vi "PSTRA-Reprocess Raw Data File.vi"(0 "Path":path, 7 "Runtime in":T1 {"window" items=["None ", "Hanning", "Hamming", "Blackman-Harris", "Exact Blackman", "Blackman", "Flat Top", "4 Term B-Harris ", "7 Term B-Harris", "Low Sidelobe"]; "stimChan"."Filter"."Stages"."IIR Filter"."Forward Coefficients" format="%.4f"; "stimChan"."Filter"."Stages"."IIR Filter"."Reverse Coefficients" format="%.4f"}, 11 "error in (no error)":errorcluster) -> (4 "Runtime out":T1 {"window" items=["None ", "Hanning", "Hamming", "Blackman-Harris", "Exact Blackman", "Blackman", "Flat Top", "4 Term B-Harris ", "7 Term B-Harris", "Low Sidelobe"]; "stimChan"."Filter"."Stages"."IIR Filter"."Forward Coefficients" format="%.4f"; "stimChan"."Filter"."Stages"."IIR Filter"."Reverse Coefficients" format="%.4f"}, 6 "PSD":dbl[][](array[numeric]), 8 "PSTH":dbl[](array[numeric]), 10 "Amplitude":dbl, 15 "error out":errorcluster)   [LabVIEW 2020]
uses:
  Typedefs/PSTR-Runtime Data.ctl
  Signal Synthesis VIs/Controls/Stimulus Channel (Full)/Full Stimulus Channel Data.ctl
  Signal Synthesis VIs/Controls/Waveform XCtl/Waveform Data.ctl
  Signal Synthesis VIs/Controls/Waveform XCtl/Waveform Enum.ctl
  Signal Synthesis VIs/Waveform VIs/Tone VIs/Tone Params.ctl
  Signal Synthesis VIs/Waveform VIs/Pulse Train VIs/Pulse Train Params.ctl
  Signal Synthesis VIs/Waveform VIs/Pulse Train VIs/Pulse Polarity.ctl
  Signal Synthesis VIs/Waveform VIs/Pulse Train VIs/PT-Continuous State.ctl
  Signal Synthesis VIs/Waveform VIs/Noise VIs/Noise Params.ctl
  Signal Synthesis VIs/Waveform VIs/File VIs/StimFile-Params.ctl
  Signal Synthesis VIs/Waveform VIs/FM Sweep VIs/FM Sweep Params.ctl
  Signal Synthesis VIs/Waveform VIs/Chirp Train VIs/Chirp Train.ctl
  Signal Synthesis VIs/Waveform VIs/Chirp Train VIs/Chirp Train Params.ctl
  Signal Synthesis VIs/Waveform VIs/Complex Tone VIs/CT-Params.ctl
  Signal Synthesis VIs/Waveform VIs/Complex Tone VIs/CT-Phase Enum.ctl
  Signal Synthesis VIs/Waveform VIs/Complex Tone VIs/CT-Runtime Data.ctl
  Signal Synthesis VIs/Waveform VIs/Moving Ripple VIs/Moving Ripple.ctl
  Signal Synthesis VIs/Waveform VIs/Moving Ripple VIs/Moving Ripple.Params.ctl
  Signal Synthesis VIs/Waveform VIs/Moving Ripple VIs/Moving Ripple.Data.ctl
  Signal Synthesis VIs/Controls/Advanced Filter XCtl/Filter Data.ctl
  Signal Synthesis VIs/Filter VIs/Filter-Bandwidth Units.ctl
  Signal Synthesis VIs/Controls/Burst XCtl/Burst Data.ctl
  Signal Synthesis VIs/Controls/Level XCtl/Level Data.ctl
  Signal Synthesis VIs/Controls/Level XCtl/Level Units.ctl
  Signal Synthesis VIs/Controls/Advanced Options XCtl/Advanced Stimulus Options.ctl
  Signal Synthesis VIs/Modulation VIs/SAM VIs/SAM Params.ctl
  <vilib>/addons/Time Series Analysis/Correlation and Spectral Analysis.llb/TSA Welch (Array).vi
  <vilib>/addons/_Advanced Signal Processing/NI_AdvSigProcTSA.lvlib
panel:
  out "reject":bool
  in  "Override":bool=TRUE
  in  "RejThr":dbl
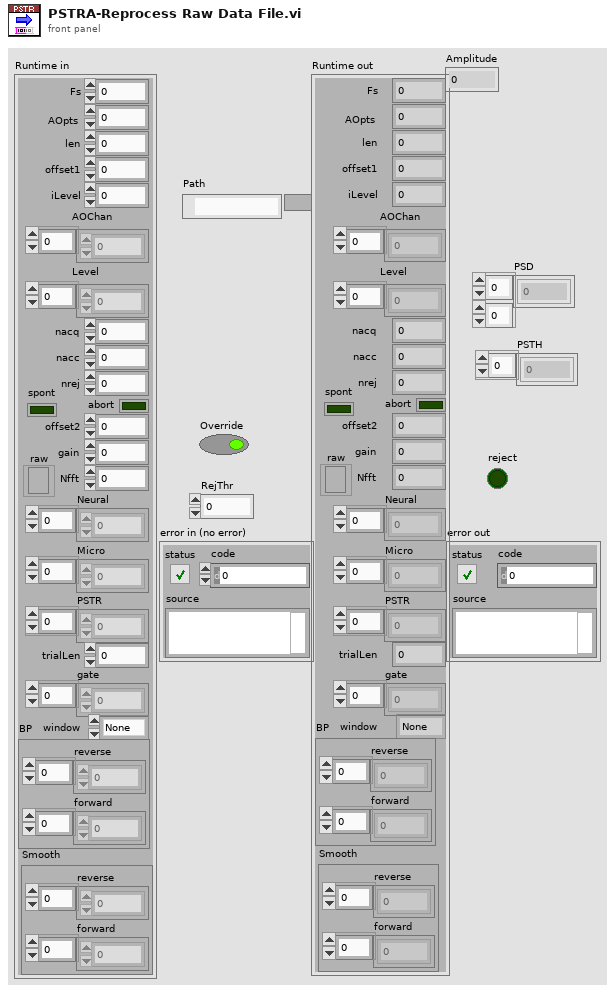
[diagram p1: front panel]
types:
  T1 = typedef "PSTR-Runtime Data.ctl" = cluster{"Fs":dbl, "AOpts":i32, "stimChan":T2, "len":i32, "offset1":i32, "iLevel":i32, "AOChan":i32[], "Level":dbl[], "nacc":i32, "nrej":i32, "nacq":i32, "abort":bool, "offset2":i32, "gain":dbl, "Nfft":i32, "Neural":dbl[], "Micro":dbl[], "raw":refnum<file>, "spont":bool, "PSTR":dbl[], "trialLen":i32, "gate":dbl[], "window":u16, "BP":cluster{"reverse":dbl[], "forward":dbl[]}, "Smooth":cluster{"reverse":dbl[], "forward":dbl[]}}
  T2 = typedef "Stimulus Channel (Full).xctl/Full Stimulus Channel Data.ctl" = cluster{"Waveform":T3, "Filter":T20, "Burst":T22, "Level":T23, "Name":string, "Advanced":T25, "SAM":T26}
  T3 = typedef "Waveform XCtl.xctl/Waveform Data.ctl" = cluster{"Type":T4, "Tone":T5, "Pulse Train":T6, "Noise":T9, "File":T10, "FMSweep":T11, "Chirp Train":T12, "Complex Tone":cluster{"Params":T14, "Data":T16}, "Moving Ripple":T17}
  T4 = typedef "Waveform Enum.ctl" = enum16{"OFF", "Tone", "Noise", "Pulse Train", "File", "FM Sweep", "Chirp Train", "Complex Tone", "FM Tone", "Moving Ripple"}
  T5 = typedef "Tone Params.ctl" = cluster{"Frequency (kHz)":dbl, "Last Freq":dbl, "Last Phase":dbl}
  T6 = typedef "Pulse Train Params.ctl" = cluster{"Pulse width (us)":dbl, "Pulse rate (Hz)":dbl, "Gap (ms)":dbl, "Polarity":T7, "PT State":T8, "Asynch":bool}
  T7 = typedef "Pulse Polarity.ctl" = enum16{"POS", "NEG", "POS-NEG", "NEG-POS"}
  T8 = typedef "PT-Continuous State.ctl" = cluster{"Template":dbl[], "Nperiod":i32, "Index":i32, "Pulse Rate (Hz)":dbl, "Phase (cycles)":dbl, "Noff":i32}
  T9 = typedef "Noise Params.ctl" = cluster{"InvFilt":bool, "Noise":dbl[], "CurPt":i32, "Aweight":bool, "Seed":i32, "afile":path}
  T10 = typedef "StimFile-Params.ctl" = cluster{"Filename":path, "Signal":dbl[], "Channel":i32, "stream":bool, "offset":i32, "nreps":i32, "loops":i32, "Randomize":bool, "order":i32[], "Seed":i32, "Tokens":i32}
  T11 = typedef "FM Sweep Params.ctl" = cluster{"Rate (oct/s)":dbl, "Fmin (Hz)":dbl, "Fmax (Hz)":dbl, "Ramp (ms)":dbl, "Linear":bool}
  T12 = typedef "Chirp Train.ctl" = cluster{"Params":T13, "Data":cluster{"WF":dbl[]}}
  T13 = typedef "Chirp Train Params.ctl" = cluster{"Fmin (kHz)":dbl, "Fmax (kHz)":dbl, "Compensate":bool, "Duration (ms)":dbl}
  T14 = typedef "CT-Params.ctl" = cluster{"F0 (Hz)":dbl, "Band":cluster{"Flow (Hz)":dbl, "Fhigh (Hz)":dbl}, "Phase":T15, "Min F0 (Hz)":dbl, "Max F0 (Hz)":dbl, "ContinRandPhase":bool, "Max peak factor":dbl, "Max mod depth":dbl, "MinHarmNum":i32, "MaxHarmNum":i32, "Level Mode":enum16{"per component", "overall rms"}, "% jitter":dbl}
  T15 = typedef "CT-Phase Enum.ctl" = enum16{"Cosine", "Random", "Alternating"}
  T16 = typedef "CT-Runtime Data.ctl" = cluster{"Ncomp":i32, "MinHarm":i32, "Phase":dbl[], "Amplitude":dbl[], "Npts/frame":i32, "Last F0":dbl, "Fmin":dbl, "Fmax":dbl, "Lslope":dbl, "randphase":bool, "overall rms":bool, "fmult":dbl[], "jittered":bool}
  T17 = typedef "Moving Ripple.ctl" = cluster{"Params":T18, "Data":T19}
  T18 = typedef "Moving Ripple.Params.ctl" = cluster{"Fmin":dbl, "Fmax":dbl, "Density":dbl, "Velocity":dbl, "Depth":dbl, "Phase":dbl, "Comp/oct":i32}
  T19 = typedef "Moving Ripple.Data.ctl" = cluster{"Freq":dbl[], "A":dbl[], "phase":dbl[], "Phase":dbl}
  T20 = typedef "Advanced Filter XCtl.xctl/Filter Data.ctl" = cluster{"Type":enum16{"Lowpass", "Highpass", "Bandpass", "Bandstop", "OFF"}, "CF (kHz)":dbl, "BW (kHz)":dbl, "Cascade":bool, "Quadrature":bool, "Scale Factor":dbl, "Stages":cluster{"IIR Filter":cluster{"filter structure":enum32{"IIR 2nd Order", "IIR 4th Order"}, "Reverse Coefficients":dbl[], "Forward Coefficients":dbl[]}, "State":dbl[]}[], "Class":enum16{"Elliptic", "Butterworth"}, "Order":i32, "BWUnits":T21}
  T21 = typedef "Filter-Bandwidth Units.ctl" = enum16{"Linear", "Octaves", "Min-Max"}
  T22 = typedef "Burst Control.xctl/Burst Data.ctl" = cluster{"Active":bool, "Delay (ms)":dbl, "Duration (ms)":dbl, "Ramp (ms)":dbl, "Rate (Hz)":dbl, "Trepeat (ms)":dbl, "Repeat":bool}
  T23 = typedef "Level XCtl.xctl/Level Data.ctl" = cluster{"Level":dbl, "Units":T24, "Max":dbl, "Multiplier":dbl, "Cal File":path, "Cal":cluster{"Freq (Hz)":dbl[], "Mag (dB SPL)":dbl[], "Phase (deg)":dbl[]}}
  T24 = typedef "Level Units.ctl" = enum16{"dB atten", "dB SPL", "dB re 1 Vrms", "dB V/Hz½", "mW", "dB HL", "Volts", "dB mW"}
  T25 = typedef "Advanced Stimulus Options.xctl/Advanced Stimulus Options.ctl" = cluster{"Rep Mask":string, "AltPol":bool, "Var":string, "Expr":string, "Persist":bool}
  T26 = typedef "SAM Params.ctl" = cluster{"Active":bool, "Frequency (Hz)":dbl, "Depth":dbl, "Init Phase (cycles)":dbl, "phase (degrees)":dbl, "Asynch":bool}
  T27 = enum16{"open", "replace", "create", "open or create", "replace or create", "replace or create with confirmation"}
  T28 = cluster{"window":u16, "length":i32, "overlap (%)":dbl}
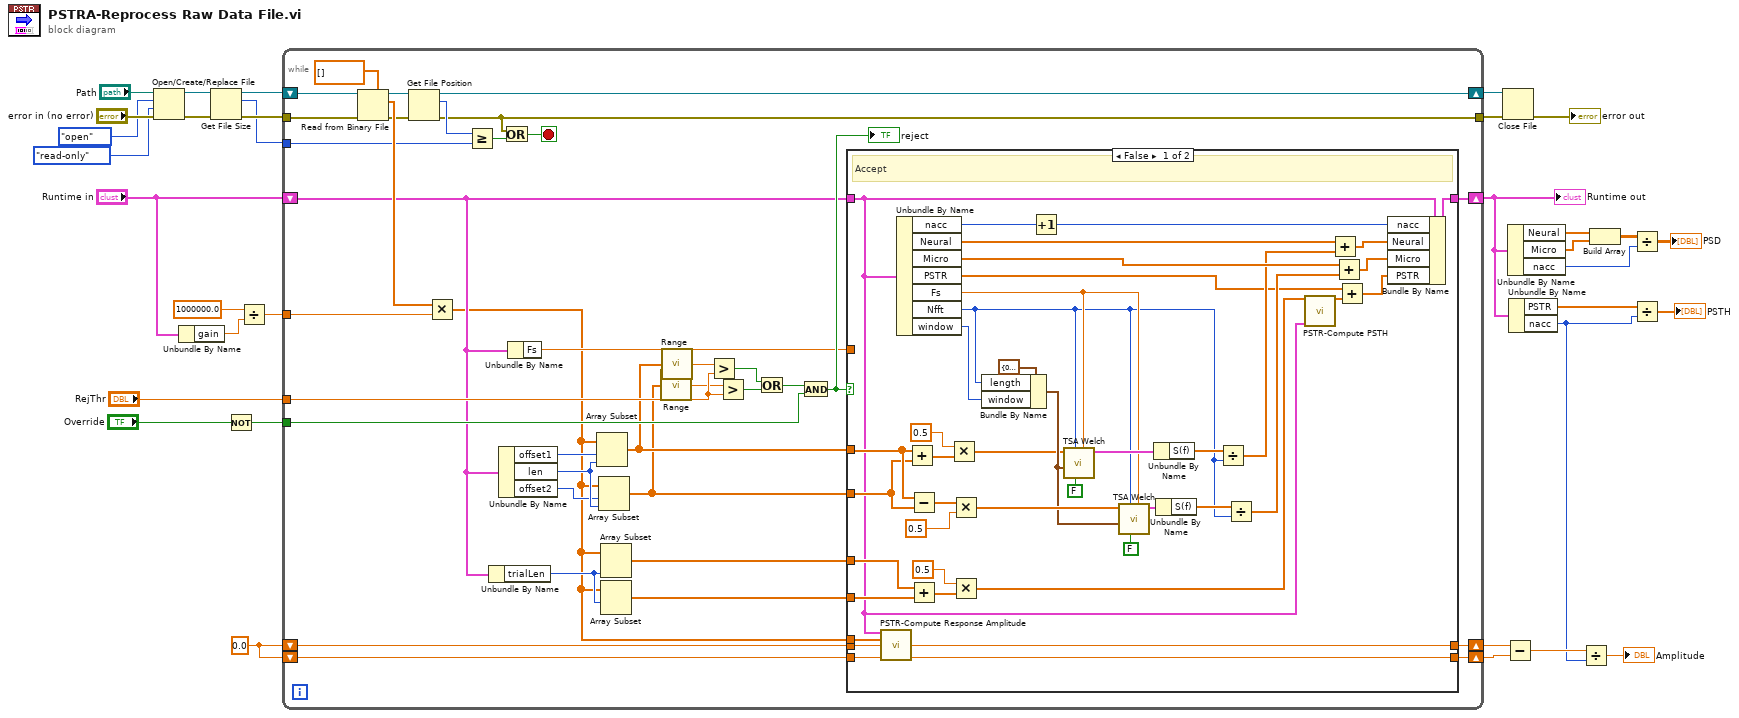
[diagram p0: block diagram]
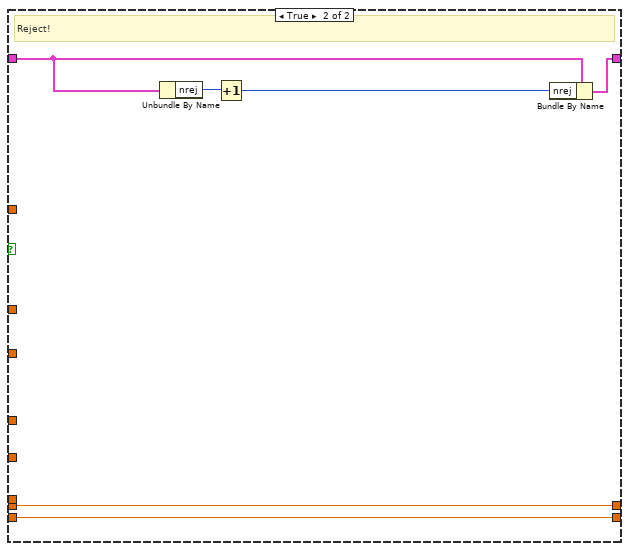
[diagram p2: hidden frame]
diagram:
  w6 = 0.0
  n1 = Open/Create/Replace File(file path (use dialog)="Path", error in="error in (no error)", operation (0:open)=T27."open", access (0:read/write)=enum16{"read/write", "read-only", "write-only"}."read-only") -> (refnum out=w23:refnum<file>, error out=w11:errorcluster)  [unwired: 2 in, 1 out]
  n2 = Unbundle By Name("Runtime in") -> ("gain"=w24:dbl)
  n3 = Get File Size(file=w23, error in=w11) -> (refnum out=w13:refnum<file>, size (in bytes)=w10:i64, 0:w12:errorcluster)
  n4 = Not(x="Override") -> (.not. x?=w30:bool)
  n5 = Divide(x=1000000.0, y=w24) -> (x/y=w22:dbl)
  n6 = while {
    tunnel: "RejThr" -> [w69]
    tunnel: w30 -> [w67]
    tunnel: w12 -> [w64]
    tunnel: w22 -> [w63]
    shift-right: [w68] -> w9
    shift-left: "Runtime in" -> [w42]
    shift-right: [w60] -> w21
    shift-left: w13 -> [w66]
    tunnel: [w47] -> w19
    tunnel: w10 -> [w49]
    shift-right: [w36] -> w5
    shift-left: w6 -> [w38]
    shift-right: [w35] -> w4
    shift-left: w6 -> [w37]
    stop <- w46 stop-if-true
    n7 = Read from Binary File(5:dbl[] [] ("data"), 8:w64, 11:w66) -> (0:w47:errorcluster, 2:w61:dbl[], 3:w62:refnum<file>)  [unwired: 3 in, 1 out]
    n8 = Get File Position(7:w62) -> (2:w50:i64, 3:w60:refnum<file>)  [unwired: 1 in, 1 out]
    n9 = Multiply(x=w61, y=w63) -> (x*y=w34:dbl[])
    n10 = Greater Or Equal?(x=w50, y=w49) -> (x >= y?=w48:bool)
    n11 = Unbundle By Name(w42) -> ("trialLen"=w39:i32)
    n12 = Unbundle By Name(w42) -> ("offset1"=w44:i32, "len"=w59:i32, "offset2"=w43:i32)
    n13 = Or(x=w47, y=w48) -> (x .or. y?=w46:bool)
    n14 = Unbundle By Name(w42) -> ("Fs"=w45:dbl)
    n15 = Array Subset(array=w34, index=w44, length=w59) -> (w52:dbl[])
    n16 = Array Subset(array=w34, index=w43, length=w59) -> (w51:dbl[])
    n17 = Array Subset(array=w34, length=w39) -> (w41:dbl[])  [unwired: 1 in]
    n18 = Array Subset(array=w34, index=w39) -> (w40:dbl[])  [unwired: 1 in]
    n19 = call "Range.vi"("Array"=w51) -> ("Range"=w57:dbl)
    n20 = call "Range.vi"("Array"=w52) -> ("Range"=w58:dbl)
    n21 = Greater?(x=w58, y=w69) -> (0:w56:bool)
    n22 = Greater?(x=w57, y=w69) -> (0:w55:bool)
    n23 = Or(x=w56, y=w55) -> (x .or. y?=w54:bool)
    n24 = And(x=w54, y=w67) -> (x .and. y?=w53:bool)
    "reject" <- w53
    n25 = case shown="False" w53 {
      tunnel: w42 -> [w70 w116]
      tunnel: [w108 w114] -> w68
      tunnel: w52 -> [w104 _]
      tunnel: w51 -> [w103 _]
      tunnel: w45 -> [_ _]
      tunnel: w41 -> [w80 _]
      tunnel: w40 -> [w79 _]
      tunnel: w38 -> [w74 w113]
      tunnel: w37 -> [w73 w112]
      tunnel: [w72 w113] -> w36
      tunnel: [w71 w112] -> w35
      tunnel: w34 -> [w75 _]
      frame False {
        # "Accept"
        n26 = call "PSTR-Compute Response Amplitude.vi"("Runtime in"=w70, "Data"=w75, "On in"=w74, "Out in"=w73) -> ("On out"=w72:dbl, "Off out"=w71:dbl)  [unwired: 10 in]
        n27 = Unbundle By Name(w70) -> ("nacc"=w109:i32, "Neural"=w95:dbl[], "Micro"=w92:dbl[], "PSTR"=w85:dbl[], "Fs"=w99:dbl, "Nfft"=w86:i32, "window"=w76:u16)
        n28 = Add(x=w104, y=w103) -> (x+y=w111:dbl[])
        n29 = Subtract(x=w104, y=w103) -> (x-y=w106:dbl[])
        n30 = Add(x=w80, y=w79) -> (x+y=w82:dbl[])
        n31 = Multiply(x=0.5, y=w111) -> (x*y=w83:dbl[])
        n32 = Multiply(x=w106, y=0.5) -> (x*y=w101:dbl[])
        n33 = Multiply(x=0.5, y=w82) -> (x*y=w78:dbl[])
        n34 = Bundle By Name(cluster=T28 {"window"=0, "length"=2048, "overlap (%)"=50.0} ("window info"), "length"=w86, "window"=w76) -> (w96:T28)
        n35 = Increment(x=w109) -> (x+1=w107:i32)
        n36 = call-poly <vilib>:"TSA Welch.vi"("sampling rate"=w99, "dB on? (T)"=FALSE, "frequency bins"=w86, "window info"=w96, "Xt"=w83) -> ("PSD"=w102:cluster{"f0":dbl, "df":dbl, "S(f)":dbl[]})  [unwired: 5 in, 1 out]
        n37 = call-poly <vilib>:"TSA Welch.vi"("sampling rate"=w99, "dB on? (T)"=FALSE, "frequency bins"=w86, "window info"=w96, "Xt"=w101) -> ("PSD"=w93:cluster{"f0":dbl, "df":dbl, "S(f)":dbl[]})  [unwired: 5 in, 1 out]
        n38 = Unbundle By Name(w102) -> ("S(f)"=w90:dbl[])
        n39 = Unbundle By Name(w93) -> ("S(f)"=w89:dbl[])
        n40 = Divide(x=w90, y=w86) -> (x/y=w88:dbl[])
        n41 = Divide(x=w89, y=w86) -> (x/y=w87:dbl[])
        n42 = call "PSTR-Compute PSTH.vi"("Signal in"=w78, "Runtime"=w70) -> ("Signal out"=w77:dbl[])  [unwired: 13 in]
        n43 = Add(x=w95, y=w88) -> (x+y=w94:dbl[])
        n44 = Add(x=w92, y=w87) -> (x+y=w91:dbl[])
        n45 = Add(x=w85, y=w77) -> (x+y=w84:dbl[])
        n46 = Bundle By Name(cluster=w70, "nacc"=w107, "Neural"=w94, "Micro"=w91, "PSTR"=w84) -> (w108:T1)
      }
      frame True {
        # "Reject!"
        n47 = Unbundle By Name(w116) -> ("nrej"=w117:i32)
        n48 = Increment(x=w117) -> (x+1=w115:i32)
        n49 = Bundle By Name(cluster=w116, "nrej"=w115) -> (w114:T1)
      }
    }
  }
  "Runtime out" <- w9
  n50 = Close File(refnum=w21, error in=w19) -> (error out=→"error out":errorcluster)  [unwired: 1 out]
  n51 = Subtract(x=w5, y=w4) -> (x-y=w3:dbl)
  n52 = Unbundle By Name(w9) -> ("Neural"=w15:dbl[], "Micro"=w16:dbl[], "nacc"=w18:i32)
  n53 = Unbundle By Name(w9) -> ("PSTR"=w8:dbl[], "nacc"=w2:i32)
  n54 = Divide(x=w3, y=w2) -> (x/y=→"Amplitude":dbl)
  n55 = Build Array(w15, w16) -> (w17:dbl[][])
  n56 = Divide(x=w17, y=w18) -> (x/y=→"PSD":dbl[][])
  n57 = Divide(x=w8, y=w2) -> (x/y=→"PSTH":dbl[])
